vi "Material-ConfigDialog-LaunchPage.vi"(0 "Configuration Dialog":refnum<class "Material-ConfigDialog.lvclass">, 5 "Configuration Page VI Filepath":path, 11 "error in":errorcluster) -> (4 "Configuration Dialog out":refnum<class "Material-ConfigDialog.lvclass">, 6 "New Navigation Tree Tag":string, 8 "Time to Launch":u32 format="%06dmsec", 15 "error out":errorcluster)   [LabVIEW 2013, in "Material-ConfigDialog.lvclass"]
uses:
  Material-ConfigDialog.lvclass
  Material-ConfigDialog.lvclass/Material-ConfigDialog.ctl
  Material-ConfigDialog-Page.ctl
  Reuse Library/featherweight/Core/Messaging/Messenger.Actor/FTW-Messenger-Actor.lvclass
panel:
  # "Inputs"
  # "Outputs"
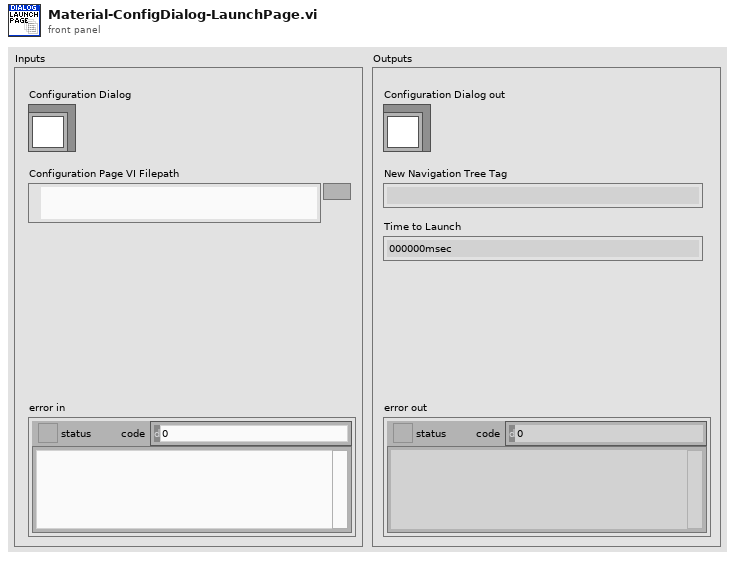
[diagram p1: front panel]
types:
  T1 = typedef "Material-ConfigDialog.lvclass/Material-ConfigDialog-Page.ctl" = cluster{"Initialized?":bool, "PageID":string, "Messenger":refnum<class "FTW-Messenger-Actor.lvclass">}
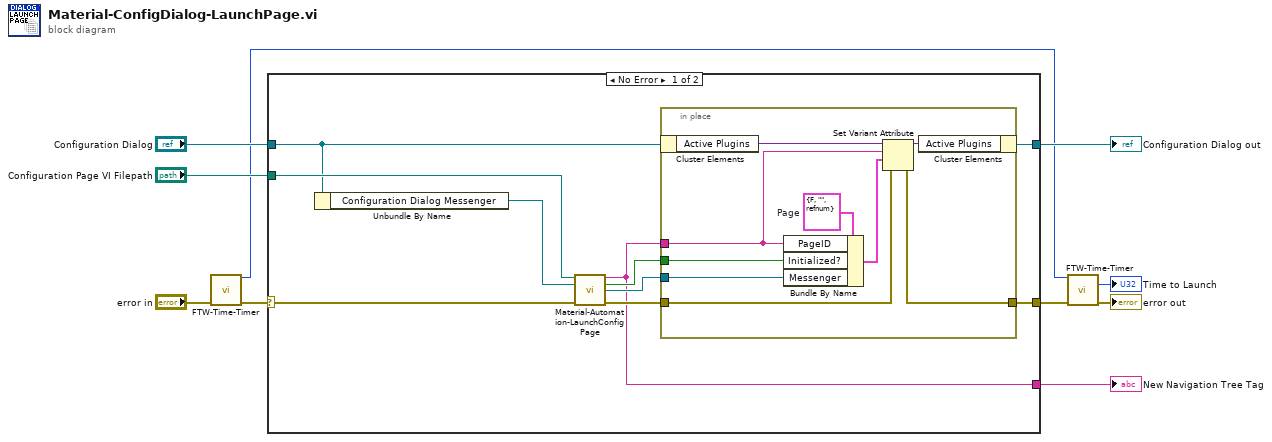
[diagram p0: block diagram]
diagram:
  n1 = call "FTW-Time-Timer.vi"("error in"="error in") -> ("Current Tick Count"=w4:u32, "error out"=w9:errorcluster)  [unwired: 12 in, 1 out]
  n2 = case shown="No Error" w9 {
    selector: w9 -> [w19 w31]
    tunnel: [w15 w31] -> w2
    tunnel: [w16 w30] -> w8
    tunnel: "Configuration Dialog" -> [w17 w30]
    tunnel: "Configuration Page VI Filepath" -> [w18 _]
    tunnel: [w11 _] -> w5
    frame No Error {
      n3 = Unbundle By Name(w17) -> ("Configuration Dialog Messenger"=w20:refnum<class "FTW-Messenger-Actor.lvclass">)
      n4 = call "Material-Automation-LaunchConfigPage.vi"("Configuration Page VI Filepath"=w18, "Config Dialog Messenger"=w20, "error in"=w19) -> ("PageID"=w11:string, "Initialized?"=w13:bool, "Page Messenger"=w12:refnum<class "FTW-Messenger-Actor.lvclass">, "error out"=w14:errorcluster)  [unwired: 9 in]
      n5 = in-place {
        in-place-border: [w24] -> w15
        in-place-border: w14 -> [w25]
        in-place-border: w13 -> [w23]
        in-place-border: w11 -> [w21]
        in-place-border: w12 -> [w22]
        w27 = T1 {"Initialized?"=FALSE, "PageID"="", "Messenger"=refnum}  # Page
        n6 = in-place-cluster #1(w17) -> ("Active Plugins"=w29:variant)
        n7 = Bundle By Name(cluster=w27, "PageID"=w21, "Initialized?"=w23, "Messenger"=w22) -> (w26:T1)
        n8 = Set Variant Attribute(Variant=w29, name=w21, value=w26, error in=w25) -> (Variant out=w28:variant, error out=w24:errorcluster)  [unwired: 1 out]
        n9 = in-place-cluster #1("Active Plugins"=w28) -> (w16:refnum<class "Material-ConfigDialog.lvclass">)
      }
    }
    frame Error {
    }
  }
  "Configuration Dialog out" <- w8
  "New Navigation Tree Tag" <- w5
  n10 = call "FTW-Time-Timer.vi"("Initial Tick Count"=w4, "error in"=w2) -> ("Elapsed Time"=→"Time to Launch":u32, "error out"=→"error out":errorcluster)  [unwired: 11 in, 1 out]
